vi "GOMDBTS2048 get Wavelength Range.vi"(8 "error in (no error)":errorcluster, 11 "handle":i32) -> (0 "error out":errorcluster, 1 "dL":dbl, 2 "L2":dbl, 3 "L1":dbl, 5 "function return":i32)   [LabVIEW 2015, in "GOMDBTS2048.lvlib"]
doc: "GOBTS2048DLL int __stdcall GOMDBTS2048_getWavelengthRange(int handle, double* L1, double* L2, double* dL);"
uses:
  GOMDBTS2048.lvlib
  runtime/GOMDBTS2048.dll
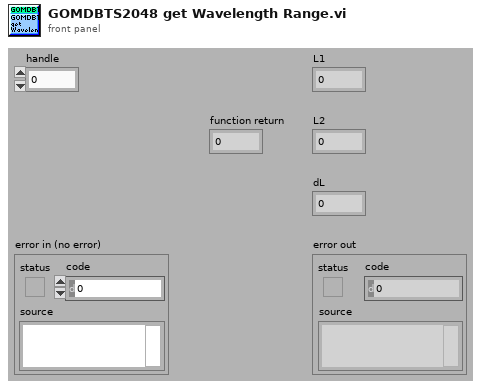
[diagram p1: front panel]
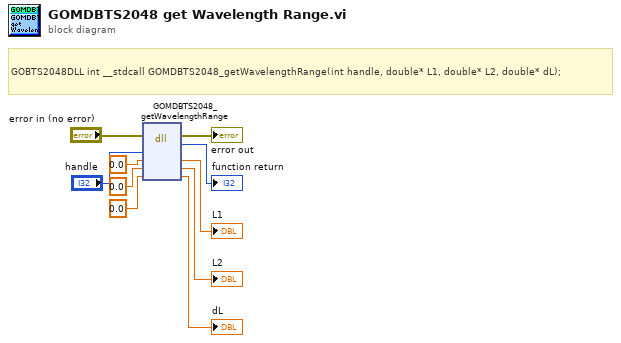
[diagram p0: block diagram]
diagram:
  # "GOBTS2048DLL int __stdcall GOMDBTS2048_getWavelengthRange(int handle, double* L1, double* L2, double* dL);"
  n1 = dll-call lib="C:/Users/rkoch/Documents/GO_Library/runtime/GOMDBTS2048.*" fn="GOMDBTS2048_getWavelengthRange"(error in="error in (no error)", "handle"="handle", "L1"=0.0, "L2"=0.0, "dL"=0.0) -> (error out=→"error out":errorcluster, →"function return":i32, "L1"=→"L1":dbl, "L2"=→"L2":dbl, "dL"=→"dL":dbl)  [unwired: 3 in, 1 out]
